vi "Straighten.vi"(6 "Bz in":dbl[](array[numeric]) format="%.5f", 8 "Error in (no error)":errorcluster, 9 "By in":dbl[](array[numeric]) format="%.5f", 10 "Bx in":dbl[](array[numeric]) format="%.5f", 11 "VISA resource":refnum<visa-resource-name>) -> (0 "Error out":errorcluster, 1 "By out":dbl[](array[numeric]) format="%.6f", 2 "Bx out":dbl[](array[numeric]) format="%.6f", 3 "Dup VISA resource":refnum<visa-resource-name>, 4 "Bz out":dbl[](array[numeric]) format="%.6f", 7 "Rotation matrix":dbl[][](array[numeric]))   [LabVIEW 2010]
doc: "Copyright (c) 2012 Metrolab Technology SA, Plan-les-Ouates, Geneva, Switzerland\nCompensate measurements for possible angular misalignments of the sensor ICs."
uses:
  <vilib>/Analysis/baseanly.llb/Real A x B.vi
  <vilib>/Analysis/NI_AALBase.lvlib
panel:
  # "Straighten"
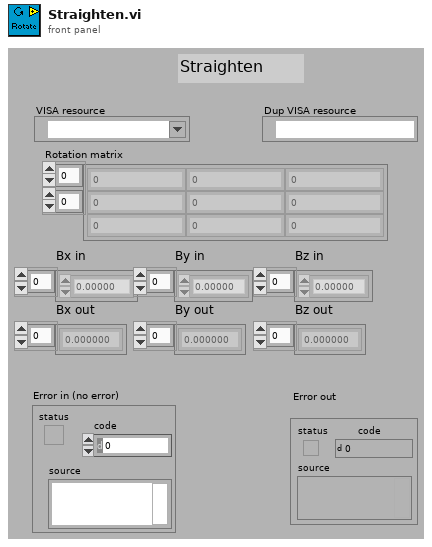
[diagram p1: front panel]
types:
  T1 = typedef "NI_Matrix.lvlib/RealMatrix.ctl" = dbl[][]
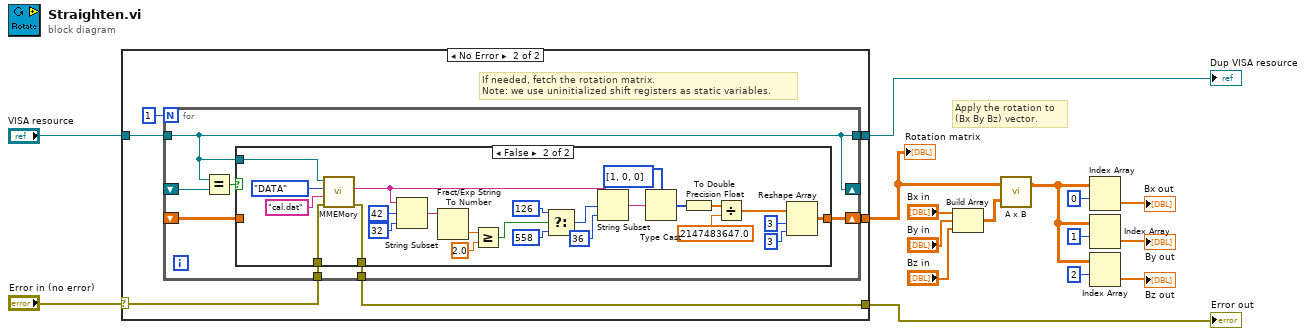
[diagram p0: block diagram]
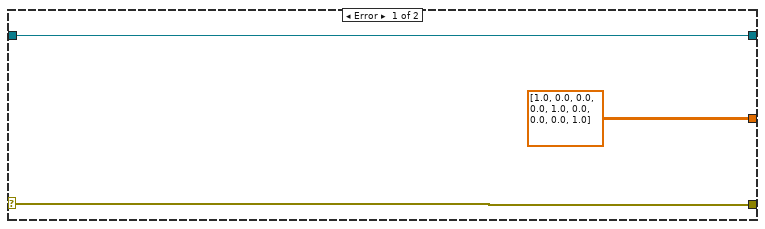
[diagram p2: hidden frame]
diagram:
  # "Apply the rotation to\n(Bx By Bz) vector."
  n1 = case shown="No Error" "Error in (no error)" {
    selector: "Error in (no error)" -> [w18 w22]
    tunnel: "VISA resource" -> [w19 w25]
    tunnel: [w19 w23] -> w13
    tunnel: [w18 w21] -> w16
    tunnel: [dbl[][] [[1.0, 0.0, 0.0], [0.0, 1.0, 0.0], [0.0, 0.0, 1.0]] w20] -> w6
    frame Error {
    }
    frame No Error {
      # "If needed, fetch the rotation matrix.\nNote: we use uninitialized shift registers as static variables."
      n2 = for {
        N: 1 -> [_]
        tunnel: w25 -> [w28]
        tunnel: w22 -> [w32]
        tunnel: [w28] -> w23
        shift-right: [w30] -> w20
        shift-left: _ -> [w31]
        shift-right: [w28] -> _
        shift-left: _ -> [w29]
        tunnel: [w27] -> w21
        n3 = Equal?(x=w28, y=w29) -> (x = y?=w26:bool)
        n4 = case shown="False" w26 {
          tunnel: w32 -> [w33 w59]
          tunnel: w31 -> [w34 _]
          tunnel: [w34 w50] -> w30
          tunnel: w28 -> [_ w48]
          tunnel: [w33 w49] -> w27
          frame True {
          }
          frame False {
            n5 = call "MMEMory.vi"("Error in (no error)"=w59, "Filename"="cal.dat", "What"=enum16{"CATalog", "DATA"}."DATA", "VISA resource"=w48) -> ("Error out"=w49:errorcluster, "Response"=w44:string)  [unwired: 5 in, 1 out]
            n6 = String Subset(string=w44, offset (0)=42, length (rest)=32 ("length (rest)")) -> (substring=w36:string)
            n7 = Fract/Exp String To Number(string=w36) -> (number=w38:dbl)  [unwired: 3 in, 1 out]
            n8 = Greater Or Equal?(x=w38, y=2.0) -> (x >= y?=w35:bool)
            n9 = Select(t=126 ("offset (0)"), s=w35, f=558 ("offset (0)")) -> (s? t:f=w41:i32)
            n10 = String Subset(string=w44, offset (0)=w41, length (rest)=36 ("length (rest)")) -> (substring=w56:string)
            n11 = Type Cast(type=i32[] [1, 0, 0], x=w56) -> (*(type *) &x=w55:i32[])
            n12 = To Double Precision Float(number=w55) -> (double precision float=w43:dbl[])
            n13 = Divide(x=w43, y=2147483647.0) -> (x/y=w53:dbl[])
            n14 = Reshape Array(w53, 3 ("dimension size"), 3 ("dimension size")) -> (w50:dbl[][])
          }
        }
      }
    }
  }
  "Error out" <- w16
  "Dup VISA resource" <- w13
  "Rotation matrix" <- w6
  n15 = Build Array("Bx in", "By in", "Bz in") -> (w5:dbl[][])
  n16 = call-poly <vilib>:"A x B.vi"("B"=w5, "A"=w6) -> ("A x B"=w4:T1)  [unwired: 1 out]
  n17 = Index Array(array=w4, index (row)=0 ("index")) -> (element=→"Bx out":dbl[])  [unwired: 1 in]
  n18 = Index Array(array=w4, index (row)=1 ("index")) -> (element=→"By out":dbl[])  [unwired: 1 in]
  n19 = Index Array(array=w4, index (row)=2 ("index")) -> (element=→"Bz out":dbl[])  [unwired: 1 in]
